vi "InitMatlabBoundControlCollection.vi"(11 "ExpID":string) -> (3 "BoundControlCollectionVariant":variant)   [LabVIEW 2017]
uses:
  MatlabGlobals.vi
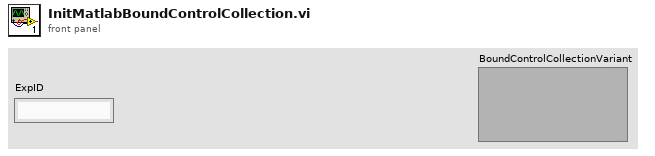
[diagram p1: front panel]
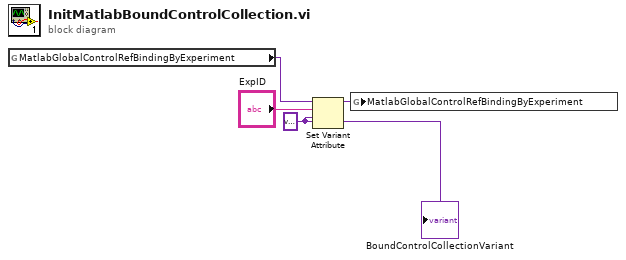
[diagram p0: block diagram]
diagram:
  w2 = variant
  n1 = global read "MatlabGlobals.vi" "MatlabGlobalControlRefBindingByExperiment"() -> (w4:variant)
  n2 = Set Variant Attribute(Variant=w4, name="ExpID", value=w2) -> (Variant out=w1:variant)  [unwired: 1 in, 2 out]
  n3 = global write "MatlabGlobals.vi" "MatlabGlobalControlRefBindingByExperiment"(w1) -> ()
  "BoundControlCollectionVariant" <- w2
